vi "CmdConsole.Read StdOut.vi"(8 "error in (no error)":errorcluster, 11 "CmdConsole in":refnum<class "CmdConsole.lvclass">) -> (0 "error out":errorcluster, 1 "Lines":string[](array[string]), 2 "Data Present":bool, 3 "CmdConsole out":refnum<class "CmdConsole.lvclass">)   [LabVIEW 2018, in "CmdConsole.lvclass"]
uses:
  CmdConsole.lvclass
  CmdConsole.lvclass/CmdConsole.ctl
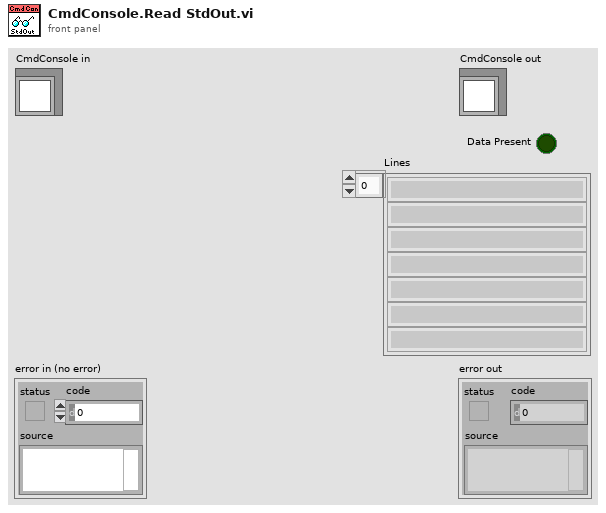
[diagram p1: front panel]
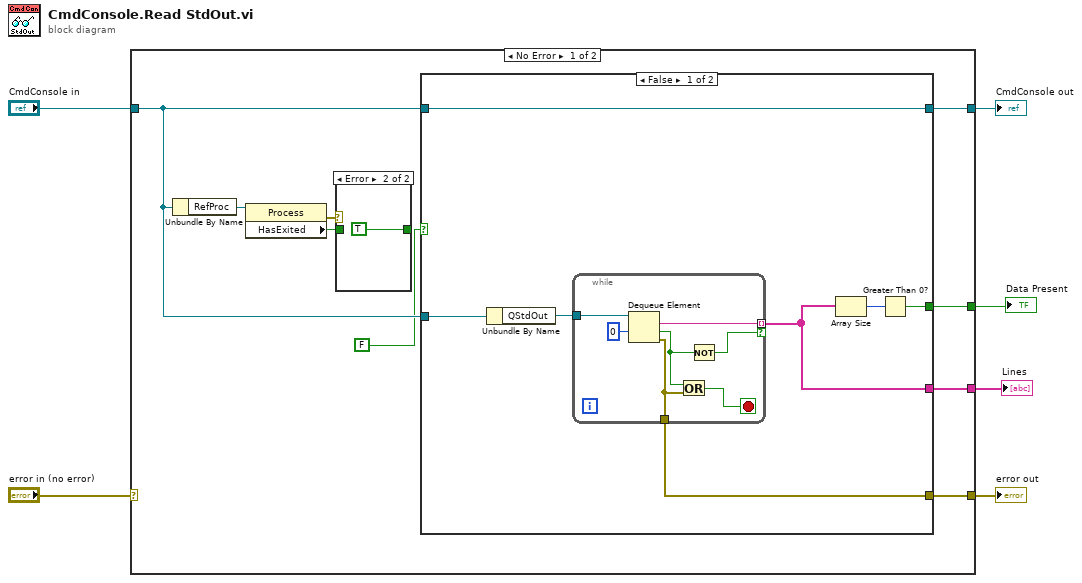
[diagram p0: block diagram]
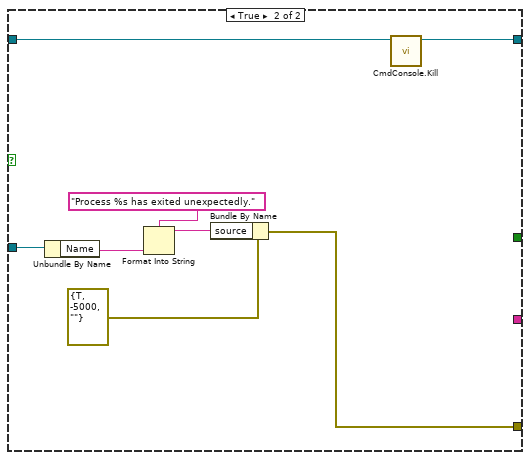
[diagram p3: hidden frame]
diagram:
  n1 = case shown="No Error" "error in (no error)" {
    selector: "error in (no error)" -> [_ w41]
    tunnel: [w12 w41] -> w5
    tunnel: [w10 w40] -> w3
    tunnel: "CmdConsole in" -> [w11 w40]
    tunnel: [w15 _] -> w2
    tunnel: [w14 _] -> w1
    frame No Error {
      n2 = Unbundle By Name(w11) -> ("RefProc"=w13:refnum<k24>)
      n3 = property class="Process"(reference=w13) -> (error out=w9:errorcluster, "HasExited"=w8:bool)  [unwired: 1 in, 1 out]
      n4 = case shown="Error" w9 {
        tunnel: w8 -> [w16 _]
        tunnel: [w16 TRUE] -> _
        frame No Error {
        }
        frame Error {
        }
      }
      n5 = case shown="False" FALSE {
        tunnel: [w23 _] -> w15
        tunnel: [w21 _] -> w14
        tunnel: w11 -> [w20 w38]
        tunnel: [w19 w34] -> w12
        tunnel: w11 -> [w18 w33]
        tunnel: [w18 w32] -> w10
        frame False {
          n6 = Unbundle By Name(w20) -> ("QStdOut"=w22:refnum<queue>)
          n7 = while {
            tunnel: w22 -> [w31]
            tunnel: [w29] -> w21 mode=indexing if=w28
            tunnel: [w25] -> w19
            stop <- w26 stop-if-true
            n8 = Dequeue Element(queue=w31, timeout in ms (-1)=0) -> (element=w29:string, timed out?=w27:bool, error out=w25:errorcluster)  [unwired: 1 in, 1 out]
            n9 = Or(x=w27, y=w25) -> (x .or. y?=w26:bool)
            n10 = Not(x=w27) -> (.not. x?=w28:bool)
          }
          n11 = Array Size(array=w21) -> (size(s)=w24:i32)
          n12 = Greater Than 0?(x=w24) -> (x > 0?=w23:bool)
        }
        frame True {
          n13 = Unbundle By Name(w38) -> ("Name"=w37:string)
          n14 = Format Into String(format string="Process %s has exited unexpectedly." ("source"), w37) -> (resulting string=w35:string)  [unwired: 2 in, 1 out]
          n15 = Bundle By Name(cluster=errorcluster {"status"=TRUE, "code"=-5000, "source"=""} ("error constant"), "source"=w35) -> (w34:errorcluster)
          n16 = call "CmdConsole.Kill.vi"("CmdConsole in"=w33) -> ("CmdConsole out"=w32:refnum<class "CmdConsole.lvclass">)  [unwired: 9 in, 1 out]
        }
      }
    }
    frame Error {
    }
  }
  "error out" <- w5
  "CmdConsole out" <- w3
  "Lines" <- w1
  "Data Present" <- w2
